vi "Read RawData.vi"(0 "VIS-NIR_STRESING_NEW in":refnum<class "VIS-NIR_STRESING_NEW.lvclass">, 5 "# of scans":i32, 9 "WCM_max_value":bool, 11 "error in (no error)":errorcluster) -> (3 "first elyse clock count":dbl, 4 "VIS-NIR_STRESING_NEW out":refnum<class "VIS-NIR_STRESING_NEW.lvclass">, 6 "Channel I":sgl[][](array[numeric]), 8 "WCM_values":T1, 10 "Channel II":sgl[][](array[numeric]), 15 "error out":errorcluster)   [LabVIEW 2020, in "VIS-NIR_STRESING_NEW.lvclass"]
uses:
  VIS-NIR_STRESING_NEW.lvclass
  C:/dev/TRANCON/Classes/GeneralFunctionality/GeneralFunctionality.lvclass
  Classes/Detector/def_repump_values_array.ctl
  Classes/Oscilloscope/def_repump_value.ctl
  Classes/GeneralFunctionality/GeneralFunctionality.lvclass/GeneralFunctionality.ctl
  <vilib>/Platform/TimedLoop/XDataNode/timing_clust.ctl
  <vilib>/Platform/TimedLoop/XDataNode/nitl_modes.ctl
  <vilib>/Platform/TimedLoop/XDataNode/wakeup.ctl
  <vilib>/platform/TimedLoop/XDataNode/XDataNode.xnode
  Classes/GeneralFunctionality/GeneralFunctionality.lvclass
  <vilib>/Platform/TimedLoop/XDataNode/XDNodeRunTimeDep.lvlib
panel:
  out "II CLEAN":i32[](graph)
  in  "Make visible":bool
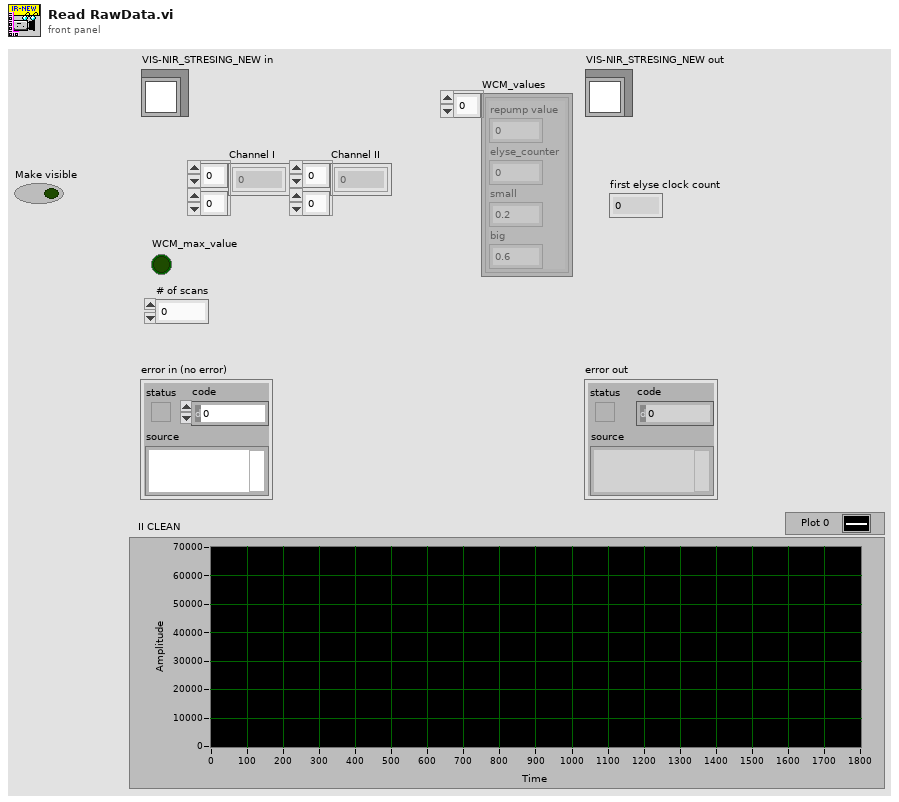
[diagram p1: front panel]
types:
  T1 = typedef "def_repump_values_array.ctl" = T2[]
  T2 = typedef "def_repump_value.ctl" = cluster{"repump value":dbl, "elyse_counter":i64, "small":dbl, "big ":dbl}
  T3 = typedef "XDNodeRunTimeDep.lvlib/timing_clust.ctl" = cluster{"Expected End [f-1]":u64, "Actual End [f-1]":u64, "Finished Late? [f-1]":bool, "Expected End [i-1]":u64, "Actual End [i-1]":u64, "Finished Late? [i-1]":bool, "Expected Start [i]":u64, "Actual Start [i]":u64, "Expected Start [f]":u64, "Actual Start [f]":u64, "Source Name":string, "Structure Name":string, "Period":i64, "Deadline":i64, "Offset":i64, "Start":i64, "Priority":i32, "Timeout":i32, "Mode":T4, "Wakeup Reason":T5, "Error":errorcluster, "Source Type":string, "Secondary Source Type":string, "Global End Time":u64, "Global Start Time":u64, "Frame Duration":u64, "Iteration Duration":u64, "Assigned CPU":i32, "I/O Scan Engine Mode":u32}
  T4 = typedef "XDNodeRunTimeDep.lvlib/nitl_modes.ctl" = enum32{"No Change", "Process missed periods, maintain original phase", "Discard missed periods, maintain original phase", "Process missed periods, ignore original phase", "Discard missed periods, ignore original phase"}
  T5 = typedef "XDNodeRunTimeDep.lvlib/wakeup.ctl" = enum32{"Normal", "Aborted", "Asynchronous wakeup", "Timing source error", "Timed loop error", "Timeout"}
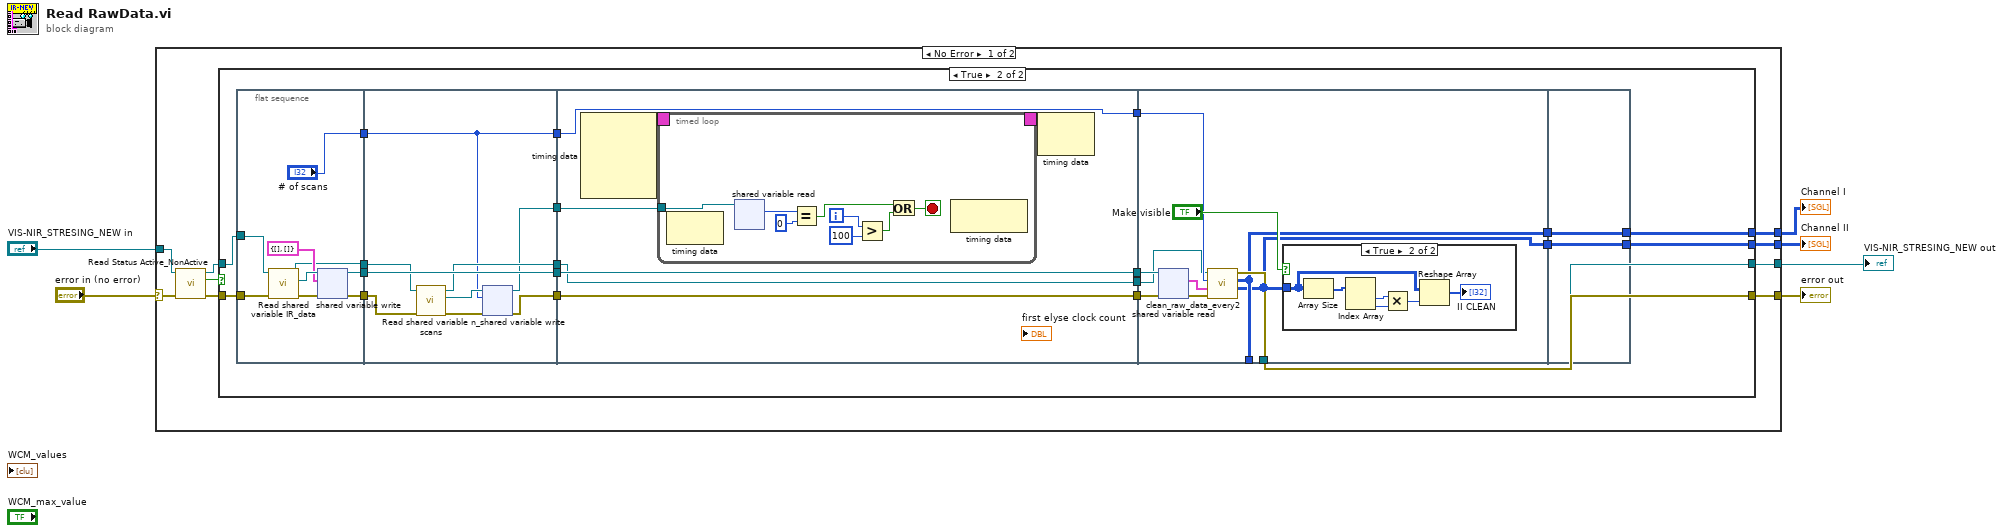
[diagram p0: block diagram]
diagram:
  n1 = case shown="No Error" "error in (no error)" {
    selector: "error in (no error)" -> [w14 w95]
    tunnel: [w7 w96] -> w3
    tunnel: "VIS-NIR_STRESING_NEW in" -> [w11 w96]
    tunnel: [w15 w95] -> w4
    tunnel: [w9 _] -> w2
    tunnel: [w8 _] -> w1
    frame No Error {
      n2 = call "Read Status Active_NonActive.vi"("error in (no error)"=w14, "GeneralFunctionality in"=w11) -> ("error out"=w13:errorcluster, "Status Active/NonActive"=w10:bool, "GeneralFunctionality out"=w12:refnum<class "VIS-NIR_STRESING_NEW.lvclass">)  [unwired: 7 in]
      n3 = case shown="True" w10 {
        tunnel: [w16 w38] -> w15
        tunnel: [w17 w33] -> w7
        tunnel: w13 -> [w16 w19]
        tunnel: w12 -> [w17 w29]
        tunnel: [_ w37] -> w9
        tunnel: [_ w34] -> w8
        frame False {
        }
        frame True {
          n4 = flat-sequence {
            tunnel: ["# of scans"] -> w27
            tunnel: [w47] -> w25
            tunnel: [w46] -> w23
            tunnel: [w42] -> w21
            tunnel: w29 -> [w41]
            tunnel: w19 -> [w39]
            tunnel: w27 -> [w48]
            tunnel: [w48] -> w26
            tunnel: w25 -> [w53]
            tunnel: [w52] -> w24
            tunnel: w23 -> [w56]
            tunnel: [w56] -> w22
            tunnel: w21 -> [w51]
            tunnel: [w50] -> w20
            tunnel: [w49] -> w18
            tunnel: [w61] -> w32
            tunnel: w26 -> [w61]
            tunnel: w24 -> [w60]
            tunnel: [w60] -> w31
            tunnel: [w59] -> w30
            tunnel: w22 -> [w59]
            tunnel: w20 -> [w58]
            tunnel: [w58] -> w28
            tunnel: w18 -> [w57]
            tunnel: [w85] -> w38
            tunnel: [w84] -> _
            tunnel: [w84] -> w36
            tunnel: [w83] -> w35
            tunnel: [w82] -> w33
            tunnel: w32 -> [w80]
            tunnel: w31 -> [w79]
            tunnel: w30 -> [w78]
            tunnel: w28 -> [w76]
            tunnel: [w94] -> w37
            tunnel: w36 -> [w94]
            tunnel: w35 -> [w93]
            tunnel: [w93] -> w34
            frame #0 {
              n5 = call-dynamic "Read shared variable IR_data.vi"("error in (no error)"=w39, "VIS-NIR_STRESING_NEW in"=w41) -> ("error out"=w43:errorcluster, "shared variable IR_data"=w45:refnum<k21>, "VIS-NIR_STRESING_NEW out"=w42:refnum<class "VIS-NIR_STRESING_NEW.lvclass">)  [unwired: 7 in]
              n6 = shared-variable-write(w45, w43, cluster{"I":i32[][], "II":i32[][]} {"I"=[], "II"=[]} ("data out")) -> (w46:refnum<k21>, w47:errorcluster)
            }
            frame #1 {
              n7 = call-dynamic "Read shared variable n_scans.vi"("error in (no error)"=w53, "VIS-NIR_STRESING_NEW in"=w51) -> ("error out"=w55:errorcluster, "shared variable n_scans"=w54:refnum<k21>, "VIS-NIR_STRESING_NEW out"=w50:refnum<class "VIS-NIR_STRESING_NEW.lvclass">)  [unwired: 7 in]
              n8 = shared-variable-write(w54, w55, w48) -> (w49:refnum<k21>, w52:errorcluster)
            }
            frame #2 {
              n9 = node-c288() -> (w63:T3)  [unwired: 4 in]
              n10 = timed-loop {
                timing: w63 -> [_]
                timing-out: [_] -> w62
                tunnel: w57 -> [w64]
                i -> [w69]
                stop <- w65 stop-if-true
                n11 = node-c288() -> ()  [unwired: 1 in, 1 out]
                n12 = shared-variable-read(w64) -> (w71:i32)  [unwired: 1 in, 3 out]
                n13 = Equal?(x=w71, y=0) -> (x = y?=w67:bool)
                n14 = Greater?(x=w69, y=100) -> (0:w66:bool)
                n15 = Or(x=w67, y=w66) -> (x .or. y?=w65:bool)
                n16 = node-c288() -> ()  [unwired: 1 in, 1 out]
              }
              n17 = node-c288(w62) -> ()  [unwired: 1 out]
            }
            frame #3 {
              n18 = shared-variable-read(w78, w79) -> (w81:errorcluster, w77:cluster{"I":i32[][], "II":i32[][]})  [unwired: 2 out]
              n19 = call-dynamic "clean_raw_data_every2.vi"("error in (no error)"=w81, "data raw"=w77, "N of scans"=w80, "VIS-NIR_STRESING_NEW in"=w76) -> ("error out"=w85:errorcluster, "I 2"=w83:i32[][], "I"=w84:i32[][], "VIS-NIR_STRESING_NEW out"=w82:refnum<class "VIS-NIR_STRESING_NEW.lvclass">)  [unwired: 4 in]
              n20 = case shown="True" "Make visible" {
                tunnel: w83 -> [_ w88]
                frame False {
                }
                frame True {
                  n21 = Array Size(array=w88) -> (size(s)=w89:i32[])
                  n22 = Index Array(array=w89) -> (element #1=w90:i32, element #2=w91:i32)  [unwired: 2 in]
                  n23 = Multiply(x=w90, y=w91) -> (x*y=w92:i32)
                  n24 = Reshape Array(w88, w92) -> (→"II CLEAN":i32[])
                }
              }
            }
            frame #4 {
            }
          }
        }
      }
    }
    frame Error {
    }
  }
  "error out" <- w4
  "VIS-NIR_STRESING_NEW out" <- w3
  "Channel II" <- w1
  "Channel I" <- w2
